vi "Get Event.vi"(8 "error in (no error)":errorcluster, 10 "id":u32, 11 "eLab in":refnum<class "PL eLabFTW Client.lvclass">) -> (0 "error out":errorcluster, 2 "event":T1 {"start datetime" format="%<%X\n%x>T"; "end datetime" format="%<%X\n%x>T"}, 3 "eLab out":refnum<class "PL eLabFTW Client.lvclass">)   [LabVIEW 2015, in "PL eLabFTW Client.lvclass"]
doc: "Gets event with the specified id."
uses:
  PL eLabFTW Client.lvclass
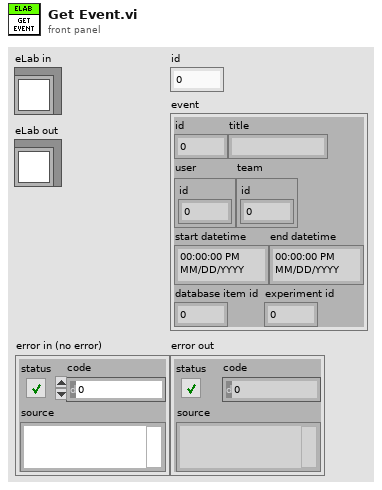
[diagram p1: front panel]
types:
  T1 = cluster{"id":u32, "title":string, "user":cluster{"id":u32}, "team":cluster{"id":u32}, "start datetime":timestamp, "end datetime":timestamp, "database item id":u32, "experiment id":u32}
  T2 = cluster{"id":string, "team":string, "item":string, "start":string, "end":string, "title":string, "userid":string, "experiment":string}
  T3 = cluster{"id":i32, "team":i32, "item":i32, "start":i32, "end":i32, "title":i32, "userid":i32, "experiment":i32}
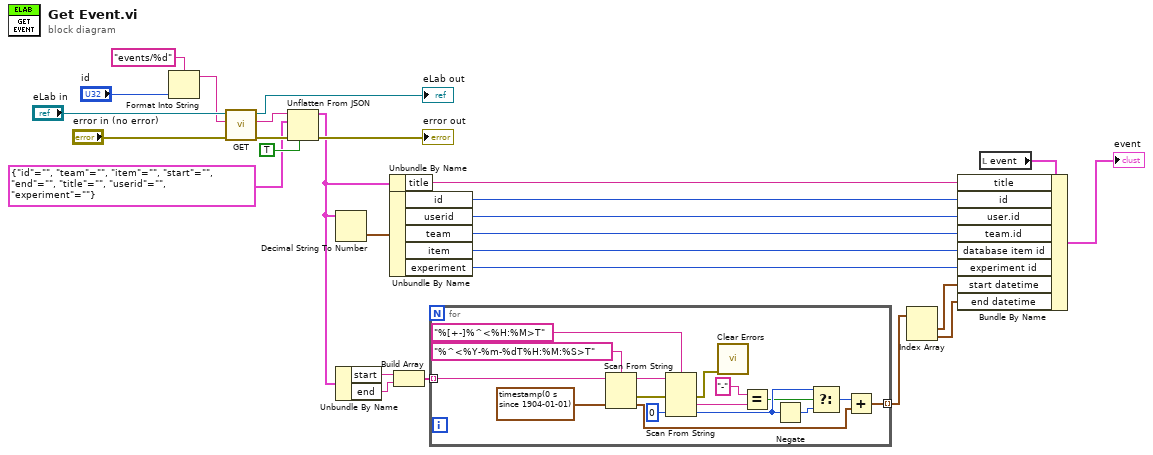
[diagram p0: block diagram]
diagram:
  n1 = Format Into String(format string="events/%d", "id") -> (resulting string=w20:string)  [unwired: 2 in, 1 out]
  n2 = call "GET.vi"("error in (no error)"="error in (no error)", "relative URL"=w20, "eLab in"="eLab in") -> ("error out"=w24:errorcluster, "response body"=w12:string, "eLab out"=→"eLab out":refnum<class "PL eLabFTW Client.lvclass">)  [unwired: 6 in]
  n3 = Unflatten From JSON(JSON string=w12, type and defaults=T2 {"id"="", "team"="", "item"="", "start"="", "end"="", "title"="", "userid"="", "experiment"=""}, default null elements? (F)=TRUE, error in (no error)=w24) -> (value=w13:T2, error out=→"error out":errorcluster)  [unwired: 3 in]
  n4 = Decimal String To Number(string=w13) -> (number=w17:T3)  [unwired: 2 in, 1 out]
  n5 = Unbundle By Name(w13) -> ("start"=w5:string, "end"=w16:string)
  n6 = Unbundle By Name(w13) -> ("title"=w18:string)
  n7 = Unbundle By Name(w17) -> ("id"=w10:i32, "userid"=w9:i32, "team"=w8:i32, "item"=w7:i32, "experiment"=w6:i32)
  n8 = Build Array(w5, w16) -> (w2:string[])
  n9 = for {
    tunnel: w2 -> [w29] mode=indexing
    tunnel: [w28] -> w1 mode=indexing
    n10 = Scan From String(format string="%^<%Y-%m-%dT%H:%M:%S>T", input string=w29, default 1=timestamp(0 s since 1904-01-01) ("default value 1")) -> (remaining string=w32:string, error out=w33:errorcluster, output 1=w40:timestamp)  [unwired: 2 in, 1 out]
    n11 = Scan From String(format string="%[+-]%^<%H:%M>T", input string=w32, error in=w33, default 2=0) -> (error out=w43:errorcluster, output 1=w36:string, output 2=w41:i32)  [unwired: 2 in, 2 out]
    n12 = call <vilib>:"Clear Errors.vi"("error in (no error)"=w43) -> ()  [unwired: 5 in, 2 out]
    n13 = Equal?(x="-", y=w36) -> (x = y?=w38:bool)
    n14 = Negate(x=w41) -> (-x=w42:i32)
    n15 = Select(t=w41, s=w38, f=w42) -> (s? t:f=w39:i32)
    n16 = Add(x=w39, y=w40) -> (x+y=w28:timestamp)
  }
  n17 = Index Array(array=w1) -> (element #1=w4:timestamp, element #2=w3:timestamp)  [unwired: 2 in]
  n18 = local read "event"() -> (w15:T1)
  n19 = Bundle By Name(cluster=w15, "title"=w18, "id"=w10, "user.id"=w9, "team.id"=w8, "database item id"=w7, "experiment id"=w6, "start datetime"=w4, "end datetime"=w3) -> (→"event":T1)
